vi "Mixed Mode Monitor.vi"() -> ()   [LabVIEW 2009]
uses:
  lib/MixedMode/Messages/Mixed Mode Status.ctl
  lib/MixedMode/Target Data.ctl
  lib/Data Access Objects/Metadata/LBCB Space.ctl
  lib/MixedMode/Mixed Mode States.ctl
  lib/MixedMode/Mixed Mode Covergance Status.ctl
  lib/MixedMode/Mixed Mode Cartesian Data.ctl
  lib/MixedMode/Stiffness Matrix.ctl
  lib/Data Access Objects/Metadata/Persistant DAO Actions.ctl
  lib/Launcher/Launcher Actions.ctl
  lib/Launcher/NoPanelAppTypes.ctl
  lib/Apps/App Status Actions.ctl
  lib/Data Access Objects/Metadata/LBCB Number.ctl
panel:
  in  "Ok":bool
  out "LBCB 2":T1=[[1000000.0, 0.0, 0.0, 0.0, 0.0, 0.0], [0.0, 1000000.0, 0.0, 0.0, 0.0, 0.0], [0.0, 0.0, 1000000.0, 0.0, 0.0, 0.0], [0.0, 0.0, 0.0, 1000000.0, 0.0, 0.0], [0.0, 0.0, 0.0, 0.0, 1000000.0, 0.0], [0.0, 0.0, 0.0, 0.0, 0.0, 1000000.0]]
  out "LBCB 1":T1=[[1000000.0, 0.0, 0.0, 0.0, 0.0, 0.0], [0.0, 1000000.0, 0.0, 0.0, 0.0, 0.0], [0.0, 0.0, 1000000.0, 0.0, 0.0, 0.0], [0.0, 0.0, 0.0, 1000000.0, 0.0, 0.0], [0.0, 0.0, 0.0, 0.0, 1000000.0, 0.0], [0.0, 0.0, 0.0, 0.0, 0.0, 1000000.0]]
  out "Mixed Mode Status Out":T2={"LBCB Target"=[], "MixedModeStates"=enum."Idle", "LBCB Convergence"=[], "LBCB Measurements"=[]}
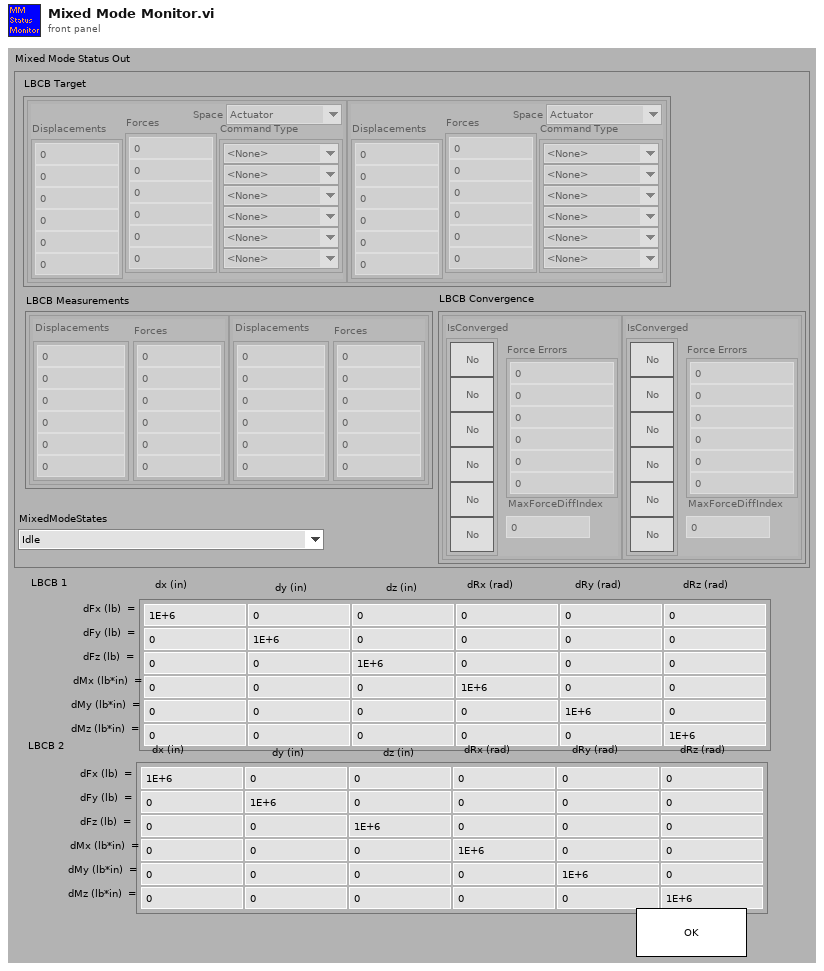
[diagram p1: front panel]
types:
  T1 = typedef "Stiffness Matrix.ctl" = dbl[][]
  T2 = typedef "Mixed Mode Status.ctl" = cluster{"LBCB Target":T3[], "MixedModeStates":T5, "LBCB Convergence":T6[], "LBCB Measurements":T7[]}
  T3 = typedef "Target Data.ctl" = cluster{"Displacements":dbl[], "Command Type":enum16{"<None>", "Displacement", "Force"}[], "Forces":dbl[], "Space":T4}
  T4 = typedef "LBCB Space.ctl" = enum16{"Actuator", "Cartesian"}
  T5 = typedef "Mixed Mode States.ctl" = enum16{"Init", "Wait For DAQ", "Idle", "Start Initial Position", "Initial Position", "Start Initial Ramp", "Run Initial Ramp", "Start Iterative Stage", "Convergence Check", "Update Stiffness Jacobian", "Update Command", "Start Iterative Ramp", "Run Iterative Ramp", "Start Iterative Stabilize", "Iterative Stabilize", "Start Iterative Holding", "Iterative Holding", "Start Stabilize", "Stabilize", "Start Hold", "Holding", "Done", "Aborting", "Exit", "Nop"}
  T6 = typedef "Mixed Mode Covergance Status.ctl" = cluster{"IsConverged":bool[], "Force Errors":dbl[], "MaxForceDiffIndex":i32}
  T7 = typedef "Mixed Mode Cartesian Data.ctl" = cluster{"Displacements":dbl[], "Forces":dbl[]}
  T8 = typedef "NoPanelAppTypes.ctl" = enum16{"NTCP Socket", "Data Archiving", "DAQ Link", "Control Loops", "Autobalance Monitor", "Mixed Mode Monitor", "Cmd Disp Diffs"}
  T9 = typedef "Launcher Actions.ctl" = enum16{"Launch", "Stop All", "Stop", "Kill", "Running?", "Init"}
  T10 = typedef "Persistant DAO Actions.ctl" = enum16{"Init", "Get", "Set", "Load", "Save"}
  T11 = typedef "App Parameters.ctl" = cluster{"Monitor Loop":T12, "Ramp Time":T12, "Log Loop":T12, "TCP to DAQ":T12, "Logging Directory":path, "Log File Size (MBytes)":i64, "Volt Logging Loop":T12}
  T12 = typedef "Timing Parameters.ctl" = cluster{"Interval":dbl, "Rate ":dbl}
  T13 = typedef "App Status Actions.ctl" = enum16{"Init", "Get Status", "Running", "Control", "Autobalanced", "Data Acquisition", "Set App State", "DAQ Started", "Set LBCB State", "Set All", "Set Cont Logging", "Set Step Logging", "Set MM Logging", "Set Volt Logging", "Set Cart Type", "Set DAQ Link", "Set NTCP Link"}
  T14 = typedef "LBCB Number.ctl" = enum16{"LBCB1", "LBCB2"}
  T15 = typedef "App Status.ctl" = cluster{"Running":bool, "Controlling L2":bool, "Autobalance L2":bool, "Data Acquisition":bool, " App State":T16, "DAQ Started":bool, "LBCB 1 State":T17, "LBCB 2 State":T17, "Controlling L1":bool, "Autobalance L1":bool, "Cartesian Type":bool, "Continuous Logging":bool, "Step Logging":bool, "Voltage Logging":bool, "Mixed Mode Logging":bool, "DAQ Link":bool, "NTCP Link ":bool}
  T16 = typedef "AppStates.ctl" = enum16{"Starting OM", "Initializing Displays", "Setting up Archiving", "Setting Up DAQ Channels", "Start DAQ", "DAQ Starting", "Controlling LBCBs", "Stopping OM"}
  T17 = typedef "Lbcb Control Loop States.ctl" = enum16{"Idle", "Start Selected", "Load Last Command", "Start Autobalancing", "Autobalancing", "Control Loop Initialized", "Control Enabled"}
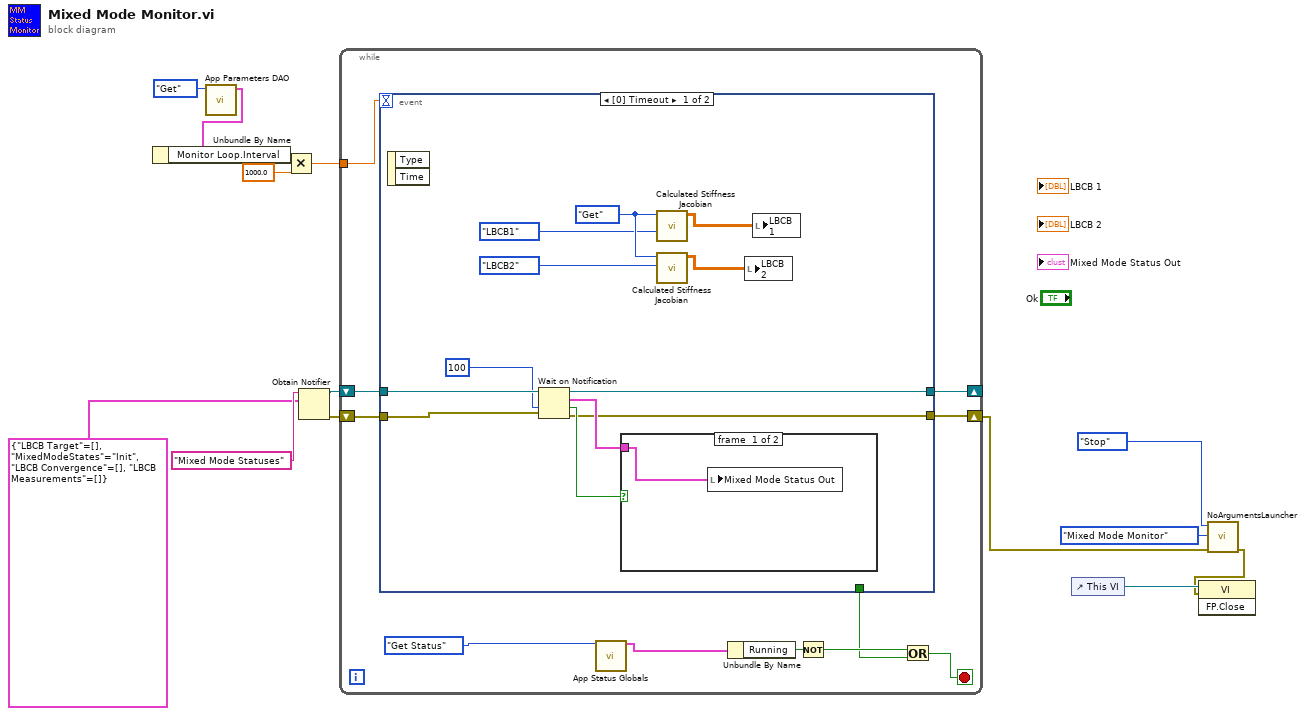
[diagram p0: block diagram]
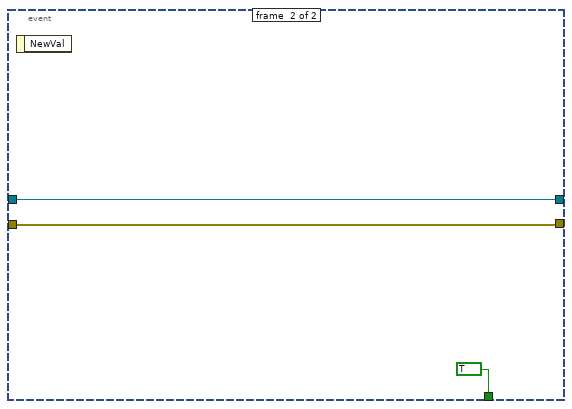
[diagram p3: hidden frame]
diagram:
  n1 = call "App Parameters DAO.vi"("Actions"=Persistant_DAO_Actions."Get") -> ("Application Timing and Logging Out"=w13:T11)  [unwired: 3 in, 7 out]
  n2 = Unbundle By Name(w13) -> ("Monitor Loop.Interval"=w12:dbl)
  n3 = Multiply(x=w12, y=1000.0) -> (x*y=w10:dbl)
  n4 = Obtain Notifier(name (unnamed)="Mixed Mode Statuses", notification data type=T2 {"LBCB Target"=[], "MixedModeStates"=enum."Init", "LBCB Convergence"=[], "LBCB Measurements"=[]} ("Mixed Mode Status")) -> (notifier out=w7:refnum<notifier>, error out=w6:errorcluster)  [unwired: 2 in, 1 out]
  n5 = while {
    tunnel: w10 -> [w20]
    shift-right: [w16] -> w3
    shift-left: w6 -> [w18]
    shift-right: [w17] -> _
    shift-left: w7 -> [w19]
    stop <- w21 stop-if-true
    n6 = event shown="[0] Timeout" {
      selector: _ -> [_ _]
      dyn-events: _ -> [_ _]
      timeout: w20 -> [_ _]
      tunnel: w19 -> [w36 w40]
      tunnel: w18 -> [w35 w39]
      tunnel: [w31 w40] -> w17
      tunnel: [w30 w39] -> w16
      tunnel: [_ TRUE] -> w15
      event #0 {
        w37 = Persistant_DAO_Actions."Get" ("Actions")
        n7 = event-data() -> ()  [unwired: 3 out]
        n8 = Wait on Notification(notifier=w36, timeout in ms (-1)=100, error in (no error)=w35) -> (notifier out=w31:refnum<notifier>, notification=w32:T2, timed out?=w33:bool, error out=w30:errorcluster)  [unwired: 1 out]
        n9 = case shown="False" w33 {
          tunnel: w32 -> [w38 _]
          frame #0 {
            n10 = local write "Mixed Mode Status Out"(w38) -> ()
          }
          frame #1 {
          }
        }
        n11 = call "Calculated Stiffness Jacobian.vi"("LBCB Number"=LBCB_Number."LBCB1", "Actions"=w37) -> ("Stiffness Jacobian Out"=w28:T1)  [unwired: 2 in, 7 out]
        n12 = call "Calculated Stiffness Jacobian.vi"("LBCB Number"=LBCB_Number."LBCB2", "Actions"=w37) -> ("Stiffness Jacobian Out"=w29:T1)  [unwired: 2 in, 7 out]
        n13 = local write "LBCB 2"(w29) -> ()
        n14 = local write "LBCB 1"(w28) -> ()
      }
      event #1 {
        n15 = event-data() -> ()  [unwired: 2 out]
      }
    }
    n16 = call "App Status Globals.vi"("App Status Actions"=App_Status_Actions."Get Status") -> ("App Status Out"=w23:T15)  [unwired: 5 in, 9 out]
    n17 = Unbundle By Name(w23) -> ("Running"=w24:bool)
    n18 = Not(x=w24) -> (.not. x?=w25:bool)
    n19 = Or(x=w25, y=w15) -> (x .or. y?=w21:bool)
  }
  n20 = control-ref of="This VI"() -> (w2:refnum<vi>)
  n21 = call "NoArgumentsLauncher.vi"("error in (no error)"=w3, "Application"=NoPanelAppTypes."Mixed Mode Monitor", "Application Launcher Actions"=Launcher_Actions."Stop") -> ("error out"=w1:errorcluster)  [unwired: 8 out]
  n22 = invoke class="VI" method="FP.Close"(reference=w2, error in=w1) -> ()  [unwired: 1 in, 3 out]
